vi "displayPlainText.vi"(8 "error in (no error)":errorcluster, 9 "Font Size":u32=70, 10 "Text In":string, 11 "TextDisplay Class in":refnum<class "TextDisplay Class.lvclass">) -> (0 "error out":errorcluster, 3 "TextDisplay Class out":refnum<class "TextDisplay Class.lvclass">)   [LabVIEW 2019, in "TextDisplay Class.lvclass"]
uses:
  TextDisplay Class.lvclass
  TextDisplay Class.lvclass/TextDisplay Class.ctl
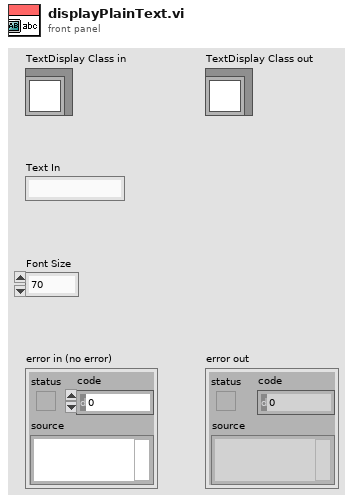
[diagram p1: front panel]
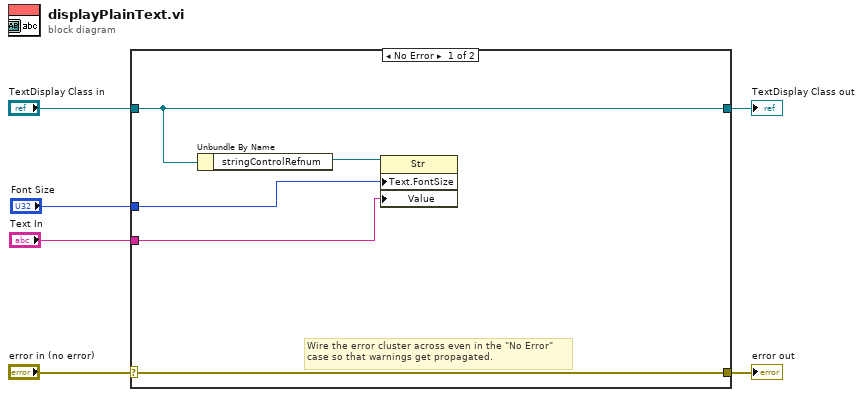
[diagram p0: block diagram]
diagram:
  n1 = case shown="No Error" "error in (no error)" {
    selector: "error in (no error)" -> [w11 w13]
    tunnel: [w11 w13] -> w5
    tunnel: [w10 w12] -> w3
    tunnel: "TextDisplay Class in" -> [w10 w12]
    tunnel: "Text In" -> [w8 _]
    tunnel: "Font Size" -> [w7 _]
    frame No Error {
      # "Wire the error cluster across even in the \"No Error\"\ncase so that warnings get propagated."
      n2 = Unbundle By Name(w10) -> ("stringControlRefnum"=w9:refnum<vi>)
      n3 = property class="Str"(reference=w9, "Text.FontSize"=w7, "Value"=w8) -> ()  [unwired: 1 in, 2 out]
    }
    frame Error {
    }
  }
  "error out" <- w5
  "TextDisplay Class out" <- w3
